vi "LS340 ReadSingalCh.vi"() -> ()   [LabVIEW 2012]
doc: "This VI was designed to demonstrate typical usage of sub vi's containing the more common 340 functions.\n\nThis example configures the loop and setpoint of the instrument, allows for a delay, and then reads sensor and heater output data. The user is given the option of just reading data and not configuring the instrument."
uses:
  <instrlib>/Lake Shore Cryotronics 340/Lake Shore Cryotronics 340.lvlib
panel:
  out "Reply":string
  in  "Configure (F:Don't Config)":bool
  in  "Delay After Config (1000 ms)":u32=1000 min=1000 max=99999 step=1
  in  "Setpoint (0.0)":dbl min=-273.0 max=300000.0 step=0.0001 format="%.4f"
  in  "Rate (D) (0)":dbl min=0.0 max=1000.0 step=1.0
  in  "Reset (I) (0.0)":dbl min=0.0 max=1000.0 step=0.1 format="%.1f"
  in  "Loop (0: 1)":u16(ring) items=["1", "2"]
  in  "Heater Range (0: Off)":u16(ring) items=["Off", "1", "2", "3", "4", "5"]
  in  "Gain (P) (0.0)":dbl min=0.0 max=1000.0 step=0.1 format="%.1f"
  in  "Manual Output (0.00)":dbl min=0.0 max=100.0 step=0.01 format="%.2f"
  out "Heater Output":dbl(slide) min=0.0 max=100.0 step=0.01 scale=0.0..100.0 scale format="%.2f"
  out "Sensor Units Reading":dbl min=-7.5 max=300000.0 step=1e-05 format="%^.5e"
  out "Kelvin Reading":dbl min=0.0 max=1645.0 step=1e-05 format="%^.5e"
  out "Celsius Reading":dbl min=-273.16 max=1372.0 step=1e-05 format="%^.5e"
  in  "Input (0: A)":u16(ring) items=["A", "B", "C", "D"]
  out "error out":errorcluster
  in  "error in (no error)":errorcluster
  in  "VISA resource name":refnum<visa-resource-name>
  # "Copyright 2005. National Instruments Corporation"
  # "Configure\nDo Not Configure"
  # "340 Temperature Controller"
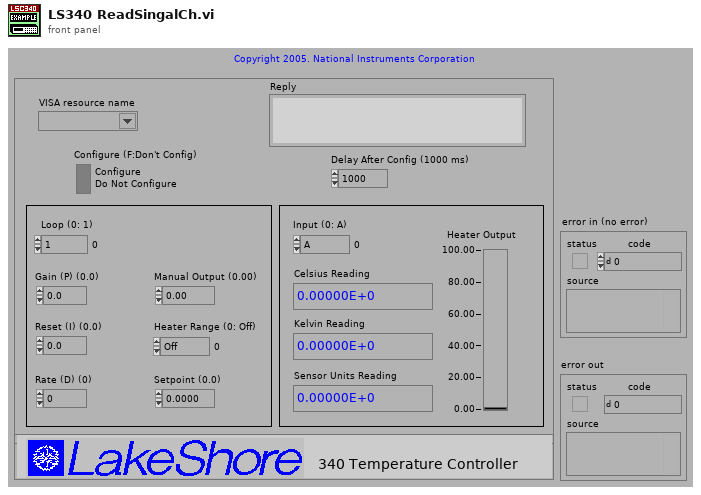
[diagram p1: front panel]
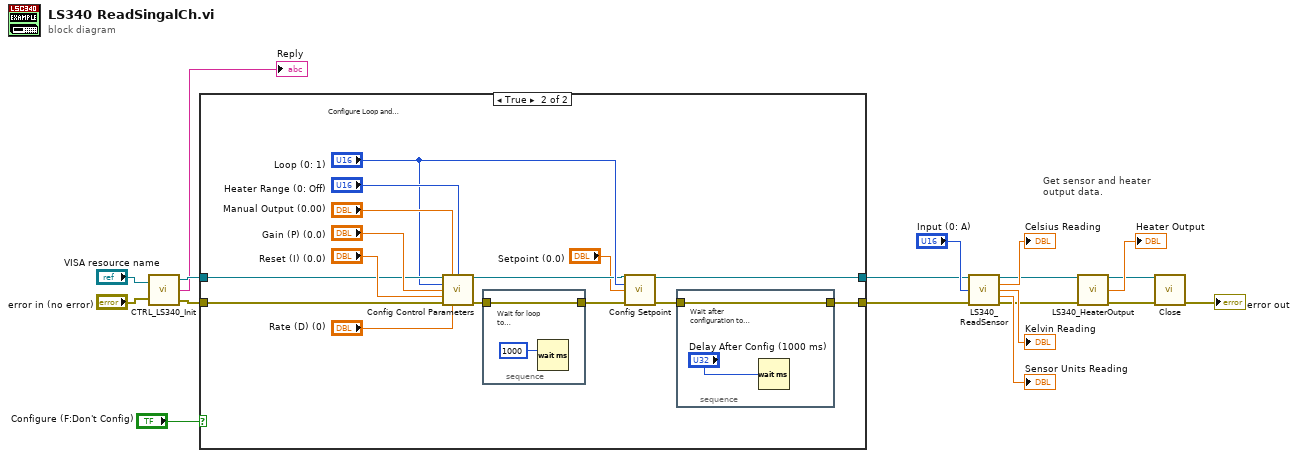
[diagram p0: block diagram]
diagram:
  # "Get sensor and heater\noutput data."
  n1 = call "CTRL_LS340_Init.vi"("error in (no error)"="error in (no error)", "found VISA"="VISA resource name") -> ("error out"=w6:errorcluster, "Reply"=→"Reply":string, "VISA Out"=w5:refnum<visa-resource-name>)
  n2 = case shown="True" "Configure (F:Don't Config)" {
    tunnel: w6 -> [w19 w35]
    tunnel: w5 -> [w20 w31]
    tunnel: [w19 w22] -> w11
    tunnel: [w20 w21] -> w10
    frame False {
      # "Do not configure Loop and Setpoint."
    }
    frame True {
      # "Configure Loop and Setpoint."
      n3 = call <instrlib>:"Config Control Parameters.vi"("VISA resource name"=w31, "Manual Output (0.00)"="Manual Output (0.00)", "Heater Range (0: Off)"="Heater Range (0: Off)", "Loop (0: 1)"="Loop (0: 1)", "Gain (P) (0.0)"="Gain (P) (0.0)", "Reset (I) (0.0)"="Reset (I) (0.0)", "error in (no error)"=w35, "Rate (D) (0)"="Rate (D) (0)") -> ("VISA resource name out"=w25:refnum<visa-resource-name>, "error out"=w28:errorcluster)  [unwired: 6 in]
      n4 = stacked-sequence {
        tunnel: w28 -> [w38]
        tunnel: [w38] -> w27
        frame #0 {
          # "Wait for loop to \nconfigure."
          n5 = Wait (ms)(milliseconds to wait=u32 1000) -> ()  [unwired: 1 out]
        }
      }
      n6 = call <instrlib>:"Config Setpoint.vi"("VISA resource name"=w25, "Loop (0: 1)"="Loop (0: 1)", "Setpoint (0.0)"="Setpoint (0.0)", "error in (no error)"=w27) -> ("VISA resource name out"=w21:refnum<visa-resource-name>, "error out"=w23:errorcluster)  [unwired: 10 in]
      n7 = stacked-sequence {
        tunnel: w23 -> [w37]
        tunnel: [w37] -> w22
        frame #0 {
          # "Wait after configuration to\nread data."
          n8 = Wait (ms)(milliseconds to wait="Delay After Config (1000 ms)") -> ()  [unwired: 1 out]
        }
      }
    }
  }
  n9 = call "LS340_ReadSensor.vi"("VISA resource name"=w10, "Input (0: A)"="Input (0: A)", "error in (no error)"=w11) -> ("VISA resource name out"=w14:refnum<visa-resource-name>, "Celsius Reading"=→"Celsius Reading":dbl, "Kelvin Reading"=→"Kelvin Reading":dbl, "Sensor Units Reading"=→"Sensor Units Reading":dbl, "error out"=w13:errorcluster)  [unwired: 8 in]
  n10 = call "LS340_HeaterOutput.vi"("VISA resource name"=w14, "error in (no error)"=w13) -> ("VISA resource name out"=w4:refnum<visa-resource-name>, "Heater Output"=→"Heater Output":dbl, "error out"=w3:errorcluster)  [unwired: 11 in]
  n11 = call <instrlib>:"Close.vi"("VISA resource name"=w4, "error in (no error)"=w3) -> ("error out"=→"error out":errorcluster)  [unwired: 13 in]
